vi "setEventId.vi"(8 "error in (no error)":errorcluster, 10 "eventId":dbl, 11 "RampEvent in":refnum<class "RampEvent.lvclass">) -> (0 "error out":errorcluster, 3 "RampEvent out":refnum<class "RampEvent.lvclass">)   [LabVIEW 2011, in "Tools.lvlib" / "Scripting.lvlib" / "RampEvent.lvclass"]
uses:
  RampEvent.lvclass
  ScriptEvent.lvclass
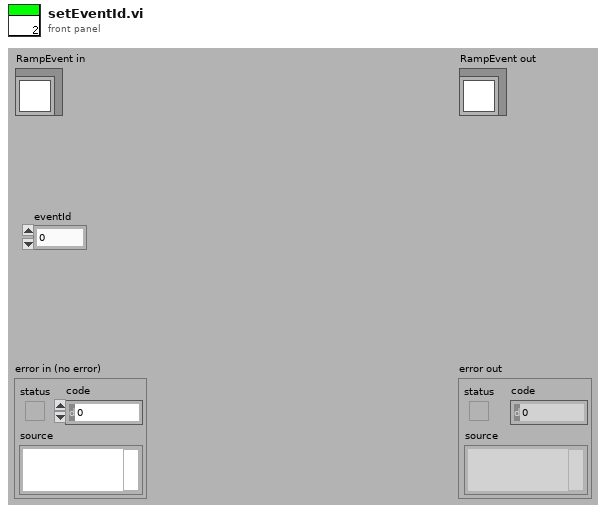
[diagram p1: front panel]
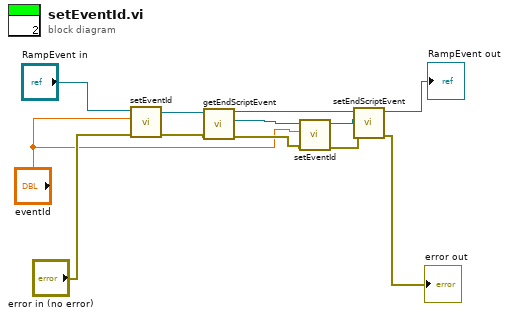
[diagram p0: block diagram]
diagram:
  n1 = call-parent "setEventId.vi"("error in (no error)"="error in (no error)", "eventId"="eventId", "ScriptEvent in"="RampEvent in") -> ("error out"=w9:errorcluster, "ScriptEvent out"=w10:refnum<class "RampEvent.lvclass">)  [unwired: 7 in]
  n2 = call "getEndScriptEvent.vi"("error in (no error)"=w9, "RampEvent.lvclass in"=w10) -> ("error out"=w4:errorcluster, "ScriptEvent.lvclass"=w2:refnum<class "ScriptEvent.lvclass">, "RampEvent.lvclass out"=w8:refnum<class "RampEvent.lvclass">)  [unwired: 7 in]
  n3 = call-dynamic "setEventId.vi"("error in (no error)"=w4, "eventId"="eventId", "ScriptEvent in"=w2) -> ("error out"=w5:errorcluster, "ScriptEvent out"=w1:refnum<class "ScriptEvent.lvclass">)  [unwired: 7 in]
  n4 = call "setEndScriptEvent.vi"("error in (no error)"=w5, "endScriptEvent.lvclass"=w1, "RampEvent.lvclass in"=w8) -> ("error out"=→"error out":errorcluster, "RampEvent.lvclass out"=→"RampEvent out":refnum<class "RampEvent.lvclass">)  [unwired: 7 in]
